vi "File Path.vi"(8 "error in (no error)":errorcluster caption="에러 입력(에러 없음)") -> (0 "error out":errorcluster caption="에러 출력", 1 "build path":path, 2 "seq":path, 3 "condition":path, 4 "경로":path)   [LabVIEW 2019]
panel:
  out "분리된 경로":path
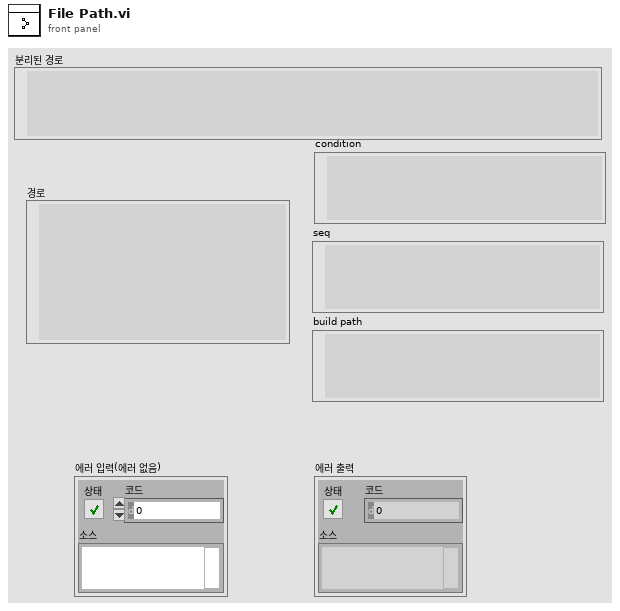
[diagram p1: front panel]
types:
  T1 = enum32{"invalid app kind", "Development System", "Run Time System", "Student Edition", "Embedded LabVIEW", "Evaluation", "Custom"}
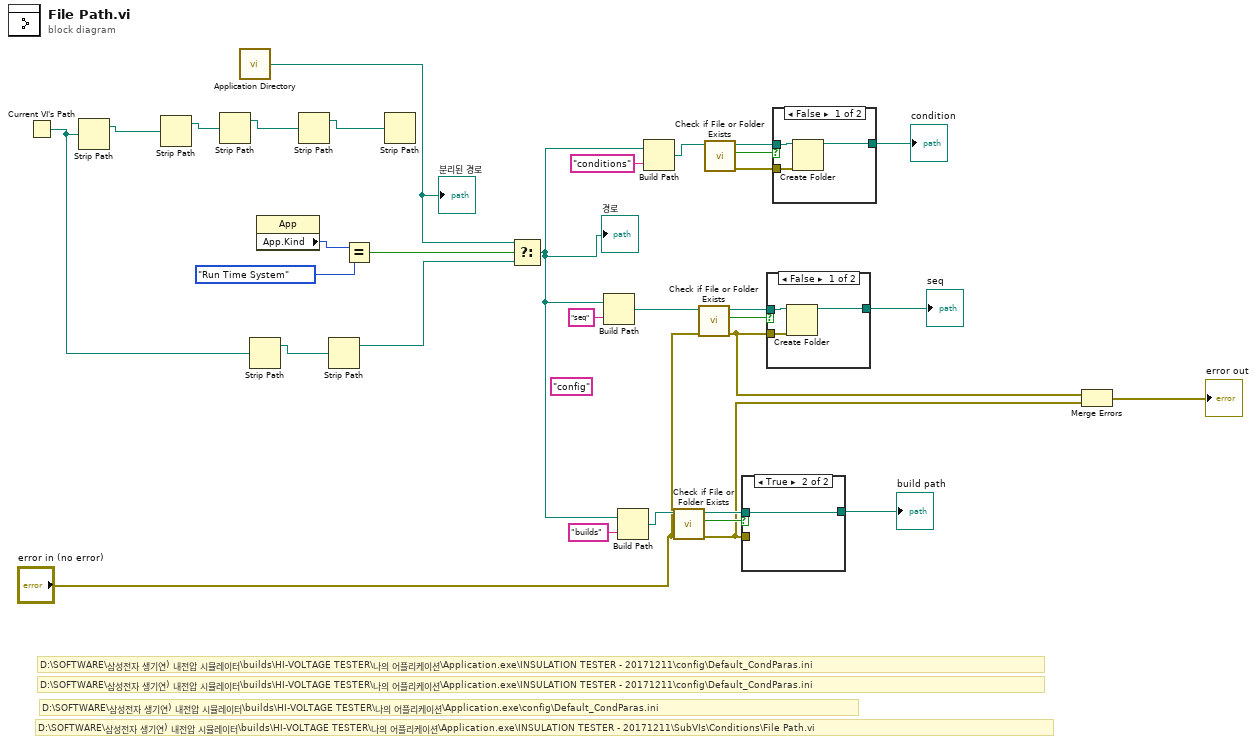
[diagram p0: block diagram]
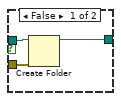
[diagram p3: hidden frame]
diagram:
  (unwired) "config" ("이름 또는 상대 경로")
  # "D:\\SOFTWARE\\삼성전자 생기연) 내전압 시뮬레이터\\builds\\HI-VOLTAGE TESTER\\나의 어플리케이션\\Application.exe\\INSULATION TESTER - 20171211\\SubVIs\\Conditions\\File Path.vi"
  # "D:\\SOFTWARE\\삼성전자 생기연) 내전압 시뮬레이터\\builds\\HI-VOLTAGE TESTER\\나의 어플리케이션\\Application.exe\\config\\Default_CondParas.ini"
  # "D:\\SOFTWARE\\삼성전자 생기연) 내전압 시뮬레이터\\builds\\HI-VOLTAGE TESTER\\나의 어플리케이션\\Application.exe\\INSULATION TESTER - 20171211\\config\\Default_CondParas.ini"
  # "D:\\SOFTWARE\\삼성전자 생기연) 내전압 시뮬레이터\\builds\\HI-VOLTAGE TESTER\\나의 어플리케이션\\Application.exe\\INSULATION TESTER - 20171211\\config\\Default_CondParas.ini"
  n1 = Current VI's Path() -> (path=w10:path)
  n2 = Strip Path(path=w10) -> (stripped path=w9:path)  [unwired: 1 out]
  n3 = Strip Path(path=w9) -> (stripped path=w11:path)  [unwired: 1 out]
  n4 = Strip Path(path=w11) -> (stripped path=w30:path)  [unwired: 1 out]
  n5 = call <vilib>:"Application Directory.vi"() -> ("Application Directory"=w8:path)
  "분리된 경로" <- w8
  n6 = Strip Path(path=w10) -> (stripped path=w27:path)  [unwired: 1 out]
  n7 = property class="App"() -> ("App.Kind"=w32:T1)  [unwired: 2 in, 2 out]
  n8 = Strip Path(path=w30) -> (stripped path=w29:path)  [unwired: 1 out]
  n9 = Strip Path(path=w27) -> (stripped path=w26:path)  [unwired: 1 out]
  n10 = Equal?(x=w32, y=T1."Run Time System") -> (x = y?=w28:bool)
  n11 = Strip Path(path=w29) -> ()  [unwired: 2 out]
  n12 = Select(t=w8, s=w28, f=w26) -> (s? t:f=w1:path)
  "경로" <- w1
  n13 = Build Path(base path=w1, name or relative path="seq" ("이름 또는 상대 경로")) -> (appended path=w23:path)
  n14 = Build Path(base path=w1, name or relative path="builds" ("이름 또는 상대 경로")) -> (appended path=w17:path)
  n15 = Build Path(base path=w1, name or relative path="conditions" ("이름 또는 상대 경로")) -> (appended path=w3:path)
  n16 = call <vilib>:"Check if File or Folder Exists.vi"("error in (no error)"="error in (no error)", "path"=w17) -> ("error out"=w13:errorcluster, "file or folder exists?"=w19:bool, "dup path"=w18:path)  [unwired: 7 in]
  n17 = call <vilib>:"Check if File or Folder Exists.vi"("error in (no error)"="error in (no error)", "path"=w23) -> ("error out"=w14:errorcluster, "file or folder exists?"=w21:bool, "dup path"=w22:path)  [unwired: 7 in]
  n18 = call <vilib>:"Check if File or Folder Exists.vi"("path"=w3) -> ("error out"=w7:errorcluster, "file or folder exists?"=w6:bool, "dup path"=w5:path)  [unwired: 8 in]
  n19 = case shown="True" w19 {
    tunnel: w18 -> [w35 w36]
    tunnel: w13 -> [w34 _]
    tunnel: [w33 w36] -> w16
    frame False {
      n20 = Create Folder(path (use dialog)=w35, error in=w34) -> (created path=w33:path)  [unwired: 1 in, 2 out]
    }
    frame True {
    }
  }
  "build path" <- w16
  n21 = case shown="False" w21 {
    tunnel: w22 -> [w39 w40]
    tunnel: w14 -> [w38 _]
    tunnel: [w37 w40] -> w20
    frame False {
      n22 = Create Folder(path (use dialog)=w39, error in=w38) -> (created path=w37:path)  [unwired: 1 in, 2 out]
    }
    frame True {
    }
  }
  "seq" <- w20
  n23 = case shown="False" w6 {
    tunnel: w5 -> [w43 w44]
    tunnel: w7 -> [w42 _]
    tunnel: [w41 w44] -> w2
    frame False {
      n24 = Create Folder(path (use dialog)=w43, error in=w42) -> (created path=w41:path)  [unwired: 1 in, 2 out]
    }
    frame True {
    }
  }
  "condition" <- w2
  n25 = Merge Errors(w14, w13) -> (→"error out":errorcluster)
